vi "IC_SetYUV2FrameHandlerSink.vi"(0 "ICImagingControl 2":refnum<k7>) -> (1 "ICImagingControl":refnum<k7>, 2 "ICImagingControl3.IFrameHandlerSink":refnum<k7>)   [LabVIEW 2020]
doc: "This VI sets IC Imaging Control's Frame Handler Sink to YUV2 pixel format. This must be used in case frame filters will be inserted in IC Imaging Control."
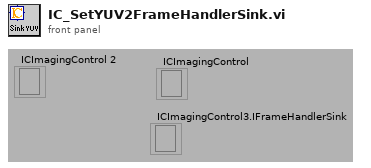
[diagram p1: front panel]
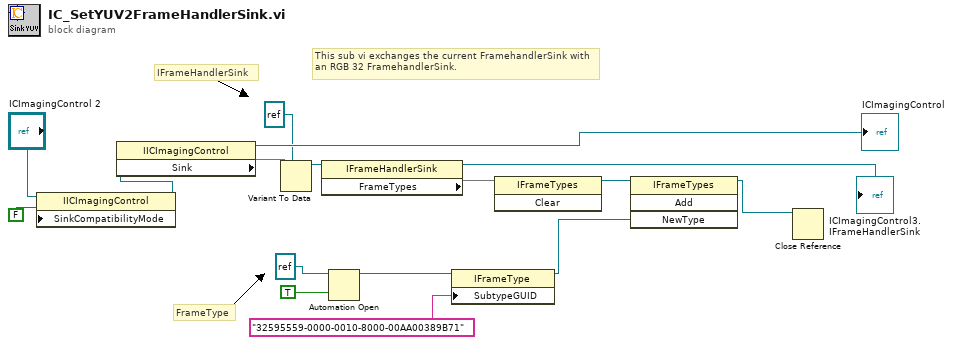
[diagram p0: block diagram]
diagram:
  # "IFrameHandlerSink"
  # "FrameType"
  # "This sub vi exchanges the current FramehandlerSink with an RGB 32 FramehandlerSink."
  n1 = property class="IICImagingControl"(reference="ICImagingControl 2", "SinkCompatibilityMode"=FALSE) -> (reference out=w3:refnum<k7>)  [unwired: 1 in, 1 out]
  n2 = property class="IICImagingControl"(reference=w3) -> (reference out=→"ICImagingControl":refnum<k7>, "Sink"=w8)  [unwired: 1 in, 1 out]
  n3 = Variant To Data(type=refnum<k7> refnum ("ICImagingControl3.IFrameHandlerSink"), Variant=w8) -> (data=w10:refnum<k7>)  [unwired: 1 in, 1 out]
  n4 = property class="IFrameHandlerSink"(reference=w10) -> (reference out=→"ICImagingControl3.IFrameHandlerSink":refnum<k7>, "FrameTypes"=w11)  [unwired: 1 in, 1 out]
  n5 = Automation Open(Automation Refnum=refnum<k7> refnum ("ICImagingControl3.IFrameType"), 9:TRUE ("open new instance")) -> (Automation Refnum=w14:refnum<k7>)  [unwired: 2 in, 1 out]
  n6 = property class="IFrameType"(reference=w14, "SubtypeGUID"="32595559-0000-0010-8000-00AA00389B71" ("Type")) -> (reference out=w6:refnum<k7>)  [unwired: 1 in, 1 out]
  n7 = invoke class="IFrameTypes" method="Clear"(reference=w11) -> (reference out=w7:refnum<k7>)  [unwired: 2 in, 2 out]
  n8 = invoke class="IFrameTypes" method="Add"(reference=w7, "NewType"=w6) -> (reference out=w5:refnum<k7>)  [unwired: 2 in, 3 out]
  n9 = Close Reference(reference=w5) -> ()  [unwired: 1 in, 1 out]
